vi "Item Add.vi"(0 "Tree Reference In":refnum<vi>, 1 "Parent Tag (Current)":string, 2 "New Tag Value (Same as Text)":string, 3 "New Text Value":string, 4 "Tree Element Data In":variant, 5 "error in (no error)":errorcluster, 6 "Child Only?":bool, 7 "Position in Branch (-1:Bottom)":i32=-1, 8 "Make Top Level Item":bool, 9 "Column Text{#1 and greater}(empty)":string[](array[string]), 11 "Symbol Index (0)":i32) -> (14 "Tree Reference Out":refnum<vi>, 16 "Created Tag":string, 19 "error out":errorcluster)   [LabVIEW 2015, in "QuickVIew.lvlib"]
doc: "Adds a new item to the tree. Uses the current selection if there is no parent value input. The tag is set to the same value as the input text if it is left blank. NOTE: TAGS MUST BE UNIQUE.TLB Prime - Application Template 1.3.0.24\nNorm Kirchner, NI Systems Engineering - NI\nCopyright (c) 2014, NI"
uses:
  QuickVIew.lvlib
  Typedef/TYPEDEF - DataStore Command.ctl
panel:
  # "VI INPUTS"
  # "VI OUTPUTS"
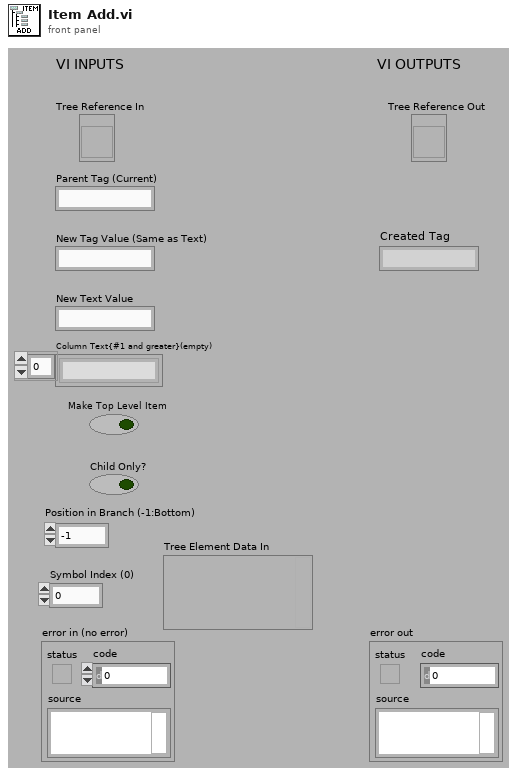
[diagram p1: front panel]
types:
  T1 = typedef "QuickVIew.lvlib/TYPEDEF - DataStore Command.ctl" = enum16{"Init", "Add", "Get", "Clear Tree", "Clear All", "Modify"}
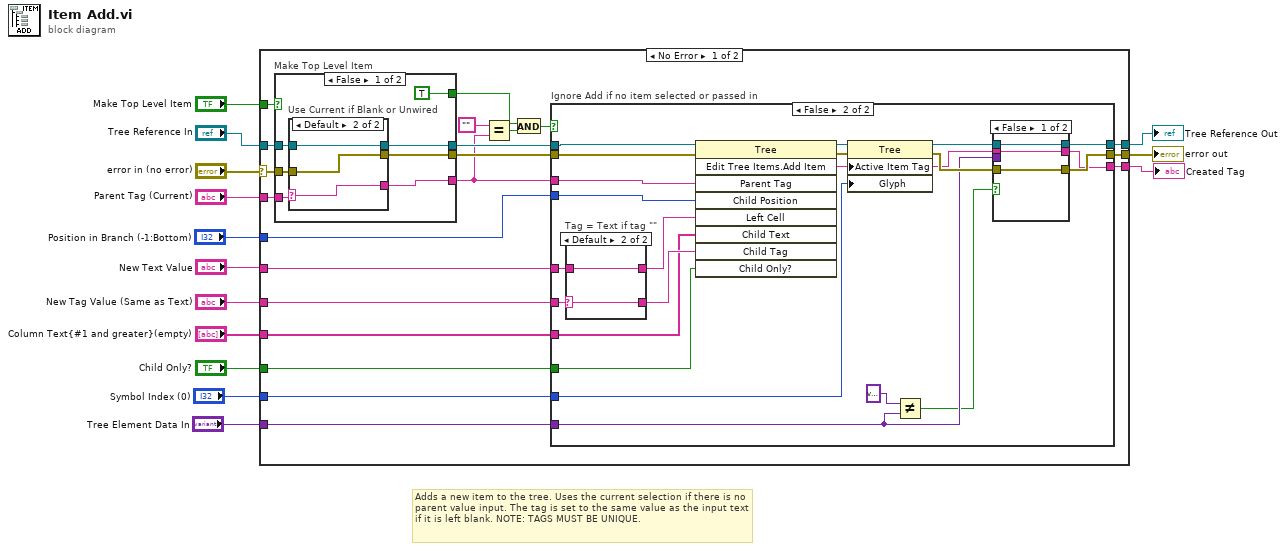
[diagram p0: block diagram]
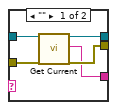
[diagram p2: hidden frame]
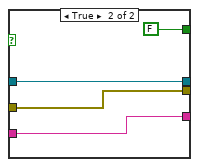
[diagram p3: hidden frame]
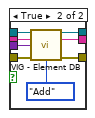
[diagram p5: hidden frame]
diagram:
  # "Adds a new item to the tree. Uses the current selection if there is no parent value input. The tag is set to the same value as the input text if it is left blank. NOTE: TAGS MUST BE UNIQUE."
  n1 = case shown="No Error" "error in (no error)" {
    selector: "error in (no error)" -> [w33 w95]
    tunnel: "Tree Reference In" -> [w35 w96]
    tunnel: [w32 w96] -> w13
    tunnel: [w31 w95] -> w12
    tunnel: "Parent Tag (Current)" -> [w34 w94]
    tunnel: "New Text Value" -> [w28 _]
    tunnel: "New Tag Value (Same as Text)" -> [w27 _]
    tunnel: "Column Text{#1 and greater}(empty)" -> [w26 _]
    tunnel: "Make Top Level Item" -> [w25 _]
    tunnel: "Child Only?" -> [w19 _]
    tunnel: [w18 w94] -> w4
    tunnel: "Position in Branch (-1:Bottom)" -> [w17 _]
    tunnel: "Symbol Index (0)" -> [w16 _]
    tunnel: "Tree Element Data In" -> [w15 _]
    frame No Error {
      n2 = case "Make Top Level Item" shown="False" w25 {
        tunnel: w35 -> [w42 w54]
        tunnel: w34 -> [w41 w52]
        tunnel: w33 -> [w40 w53]
        tunnel: [w39 w54] -> w30
        tunnel: [w38 w53] -> w29
        tunnel: [w37 w52] -> w21
        tunnel: [TRUE FALSE] -> w22
        frame False {
          n3 = case "Use Current if Blank or Unwired" shown="Default" w41 {
            selector: w41 -> [_ w48]
            tunnel: [w46 w50] -> w39
            tunnel: w42 -> [w47 w50]
            tunnel: [w45 w49] -> w38
            tunnel: w40 -> [w44 w49]
            tunnel: [w43 w48] -> w37
            frame "" {
              n4 = call "Get Current.vi"("Tree Reference In"=w47, "error in (no error)"=w44) -> ("Tree Reference Out"=w46:refnum<vi>, "Current Tag"=w43:string, "error out"=w45:errorcluster)  [unwired: 15 out]
            }
            frame Default {
            }
          }
        }
        frame True {
        }
      }
      n5 = Equal?(x="", y=w21) -> (x = y?=w23:bool)
      n6 = And(x=w22, y=w23) -> (x .and. y?=w20:bool)
      n7 = case "Ignore Add if no item selected or passed in" shown="False" w20 {
        tunnel: [w57 w66] -> w32
        tunnel: [w56 w64] -> w31
        tunnel: w30 -> [w57 w77]
        tunnel: w29 -> [w56 w76]
        tunnel: w28 -> [_ w78]
        tunnel: w27 -> [_ w79]
        tunnel: w26 -> [_ w71]
        tunnel: w21 -> [w55 w73]
        tunnel: w19 -> [_ w70]
        tunnel: [w55 w62] -> w18
        tunnel: w17 -> [_ w72]
        tunnel: w16 -> [_ w67]
        tunnel: w15 -> [_ w60]
        frame True {
        }
        frame False {
          n8 = case "Tag = Text if tag \"\"" shown="Default" w79 {
            selector: w79 -> [_ w92]
            tunnel: w78 -> [w91 w93]
            tunnel: [w91 w93] -> w75
            tunnel: [w91 w92] -> w74
            frame "" {
            }
            frame Default {
            }
          }
          n9 = invoke class="Tree" method="Edit Tree Items.Add Item"(reference=w77, error in=w76, "Parent Tag"=w73, "Child Position"=w72, "Left Cell"=w75, "Child Text"=w71, "Child Tag"=w74, "Child Only?"=w70) -> (reference out=w68:refnum<vi>, error out=w69:errorcluster, "Edit Tree Items:Add Item"=w63:string)  [unwired: 1 in, 6 out]
          n10 = property class="Tree"(reference=w68, error in=w69, "Active Item Tag"=w63, "Glyph"=w67) -> (reference out=w61:refnum<vi>, error out=w65:errorcluster)
          n11 = Not Equal?(x=variant ("Tree Element Data In"), y=w60) -> (x != y?=w58:bool)
          n12 = case shown="False" w58 {
            tunnel: [w81 w90] -> w66
            tunnel: w65 -> [w82 w89]
            tunnel: [w82 w88] -> w64
            tunnel: w63 -> [w80 w86]
            tunnel: [w80 w85] -> w62
            tunnel: w61 -> [w81 w84]
            tunnel: w60 -> [_ w83]
            frame False {
            }
            frame True {
              n13 = call "VIG - Element DB.vi"("Tree Ref In"=w84, "Element Tag"=w86, "Tree Element Data In"=w83, "error in (no error)"=w89, "Command"=TYPEDEF_-_DataStore_Command."Add") -> ("Tree Ref Out"=w90:refnum<vi>, "Element Tag Out"=w85:string, "error out"=w88:errorcluster)  [unwired: 8 out]
            }
          }
        }
      }
    }
    frame Error {
    }
  }
  "Tree Reference Out" <- w13
  "error out" <- w12
  "Created Tag" <- w4
